vi "Obtener TemperaturaBalero DB.vi"(8 "error in (no error)":errorcluster) -> (0 "error out":errorcluster, 3 "TEMPERATURABALERO":dbl[](array[numeric]))   [LabVIEW 2020]
uses:
  <vilib>/drjdpowell/SQLite Library/SQL Connection/Open (path).vi
  <vilib>/drjdpowell/SQLite Library/SQL Connection/Open (string).vi
  <vilib>/AdvancedString/Path To Command Line String.vi
  <vilib>/drjdpowell/SQLite Library/SQL Connection/Execute SQL (1D DBL results).vi
  <vilib>/drjdpowell/SQLite Library/SQL Connection/Connection.lvclass
  DataBaseSQLlite.lvlib
  <vilib>/drjdpowell/SQLite Library/SQLite.lvlib
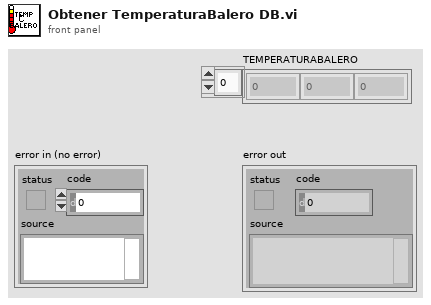
[diagram p1: front panel]
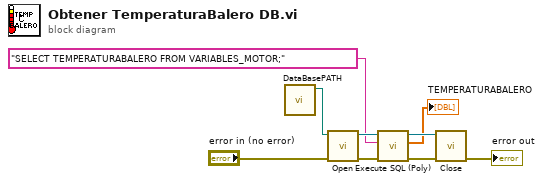
[diagram p0: block diagram]
diagram:
  n1 = call "DataBasePATH.vi"() -> ("DataBase path"=w9:path)  [unwired: 11 in]
  n2 = call-poly <vilib>:"Open.vi"("error in (no error)"="error in (no error)", "db file"=w9) -> ("error out"=w6:errorcluster, "SQLite Connection"=w7:refnum<class "Connection.lvclass">)  [unwired: 8 in]
  n3 = call-poly <vilib>:"Execute SQL (Poly).vi"("error in (no error)"=w6, "SQL"="SELECT TEMPERATURABALERO FROM VARIABLES_MOTOR;", "SQLite Connection in"=w7) -> ("error out"=w3:errorcluster, "Result Set"=→"TEMPERATURABALERO":dbl[], "SQLite Connection"=w4:refnum<class "Connection.lvclass">)  [unwired: 5 in, 1 out]
  n4 = call-dynamic "Close.vi"("error in (no error)"=w3, "SQLite Connection in"=w4) -> ("error out"=→"error out":errorcluster)  [unwired: 9 in]
